vi "PNG Header.vi"(0 "Path In":path, 1 "Mode":u16(ring)=1 items=["Write", "read"], 5 "Path Out":path, 7 "header in":string="ROI", 9 "string in":string, 11 "error in (no error)":errorcluster, 12 "index (-1 last entry)":i32=-1) -> (4 "pathOut":path, 6 "Actual Index":i32, 8 "header out":string, 10 "string out":string, 15 "error out":errorcluster)   [LabVIEW 2009, in "POLARIS Vision utility.lvlib"]
doc: "This VI allow you to store custom strings in a PNG file. It supports storing multiple strings at various indexes starting with 0. Each index contains a header (max of 64 characters), and the text (no size limit). These could be used to have the header say \"Patient's name\" and the text have \"John Doe\" for example. You could also save data acqusition to a image file by using the FlattenToString.vi to compress the data into a string, and then uncompress it later. If you specify an index to read or write that is out of range, the function will return the last entry's index, this way you can find out how many text entries are in the file.\n\nIf no Path Out is specified, the Path In is used to save the data to. In Read Mode, the Header In and Text In are ignored. If you try to read from a PNG with no embedded text, the returned index will be -1."
uses:
  POLARIS Vision utility.lvlib
  NI_PNGCustomString.dll
panel:
  # "Max of ~64"
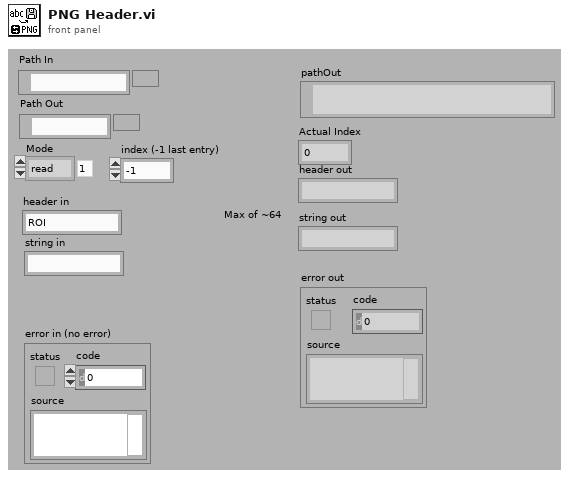
[diagram p1: front panel]
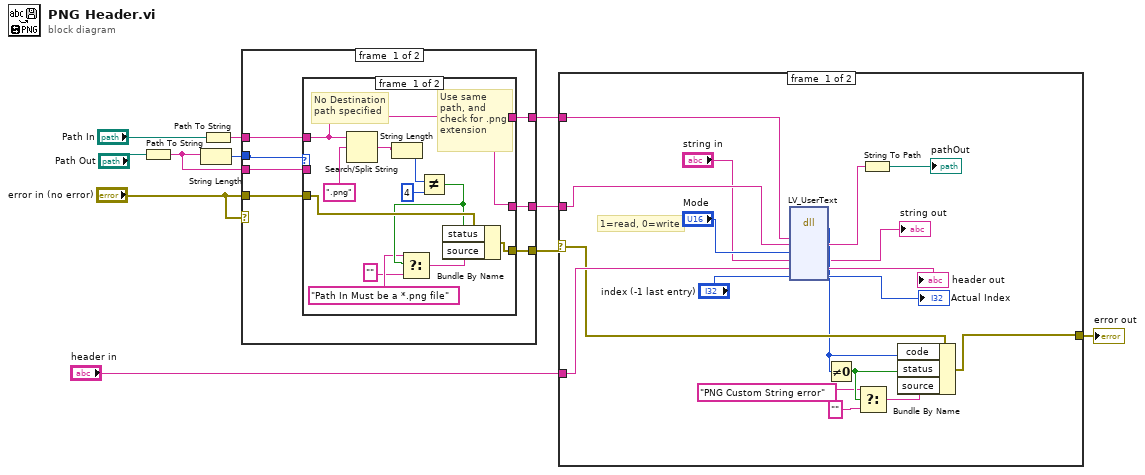
[diagram p0: block diagram]
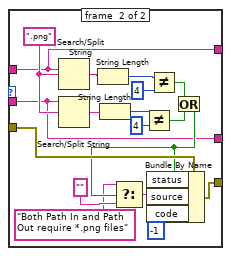
[diagram p2: hidden frame]
diagram:
  n1 = Path To String(path="Path Out") -> (string=w7:string)
  n2 = String Length(string=w7) -> (length=w10:i32)
  n3 = Path To String(path="Path In") -> (string=w9:string)
  n4 = case shown="No Error" "error in (no error)" {
    selector: "error in (no error)" -> [_ w50]
    tunnel: w10 -> [w18 _]
    tunnel: "error in (no error)" -> [w17 _]
    tunnel: w9 -> [w16 w49]
    tunnel: [w15 w50] -> w8
    tunnel: w7 -> [w14 w48]
    tunnel: [w13 w49] -> w6
    tunnel: [w12 w48] -> w5
    frame #0 {
      n5 = case shown="1, Default" w18 {
        tunnel: w17 -> [w25 w38]
        tunnel: w16 -> [w22 w35]
        tunnel: [w24 w37] -> w15
        tunnel: w14 -> [_ w34]
        tunnel: [w22 w35] -> w13
        tunnel: [w22 w34] -> w12
        frame #0 {
          # "No Destination path specified"
          # "Use same path, and check for .png extension"
          n6 = Search/Split String(string=w22, search string/char (-)=".png") -> (match + rest of string=w28:string)  [unwired: 1 in, 2 out]
          n7 = String Length(string=w28) -> (length=w27:i32)
          n8 = Not Equal?(x=w27, y=4) -> (x != y?=w23:bool)
          n9 = Select(t="Path In Must be a *.png file" ("source"), s=w23, f="" ("t")) -> (s? t:f=w21:string)
          n10 = Bundle By Name(cluster=w25, "status"=w23, "source"=w21) -> (w24:errorcluster)
        }
        frame #1 {
          w47 = ".png"
          n11 = Search/Split String(string=w35, search string/char (-)=w47) -> (match + rest of string=w45:string)  [unwired: 1 in, 2 out]
          n12 = Search/Split String(string=w34, search string/char (-)=w47) -> (match + rest of string=w46:string)  [unwired: 1 in, 2 out]
          n13 = String Length(string=w45) -> (length=w41:i32)
          n14 = String Length(string=w46) -> (length=w42:i32)
          n15 = Not Equal?(x=w42, y=4) -> (x != y?=w39:bool)
          n16 = Not Equal?(x=w41, y=4) -> (x != y?=w40:bool)
          n17 = Or(x=w40, y=w39) -> (x .or. y?=w36:bool)
          n18 = Select(t="Both Path In and Path Out require *.png files", s=w36, f="" ("t")) -> (s? t:f=w33:string)
          n19 = Bundle By Name(cluster=w38, "status"=w36, "source"=w33, "code"=-1) -> (w37:errorcluster)
        }
      }
    }
    frame #1 {
    }
  }
  n20 = case shown="No Error" w8 {
    selector: w8 -> [w59 w69]
    tunnel: w6 -> [w62 _]
    tunnel: w5 -> [w61 _]
    tunnel: [w58 w69] -> w4
    tunnel: "header in" -> [w60 _]
    frame #0 {
      # "1=read, 0=write"
      n21 = dll-call lib="D:/POLARIS Vision/Utility/Write PNG Header/NI_PNGCustomString.dll" fn="LV_UserText"("pathIn"=w62, "pathOut"=w61, "mode"="Mode", "text"="string in", "header"=w60, "index"="index (-1 last entry)") -> (w57:i32, "pathOut"=w65:string, "text"=→"string out":string, "header"=→"header out":string, "index"=→"Actual Index":i32)  [unwired: 5 in, 2 out]
      n22 = Not Equal To 0?(x=w57) -> (x != 0?=w56:bool)
      n23 = Select(t="PNG Custom String error", s=w56, f="") -> (s? t:f=w53:string)
      n24 = String To Path(string=w65) -> (path=→"pathOut":path)
      n25 = Bundle By Name(cluster=w59, "code"=w57, "status"=w56, "source"=w53) -> (w58:errorcluster)
    }
    frame #1 {
    }
  }
  "error out" <- w4
